vi "TestProgram_SingleStep.vi"() -> ()   [LabVIEW 2011]
uses:
  <instrlib>/Newport ESP301/Newport ESP301.lvlib
panel:
  out "x-y":dbl(graph)
  out "Reduction Ratio":dbl format="%.6g"
  out "Power Status":bool
  out "error out 2":errorcluster
  out "Velocity (units/s)":dbl format="%.4g"
  out "Position (units)":dbl(graph)
  in  "Axis (1)":i32=1
  out "DAC Offset":dbl format="%.6g"
  out "error out":errorcluster
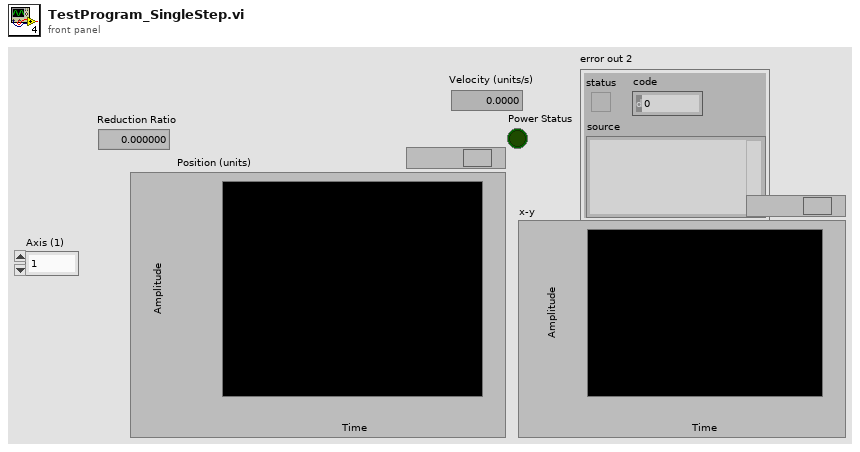
[diagram p1: front panel]
types:
  T1 = enum16{"Trapezoidal Mode", "S-curve Mode", "Jog Mode", "Slave to master's desired position (trajectory)", "Slave to master's actual position (feedback)", "Slave to master's actual velocity for jogging"}
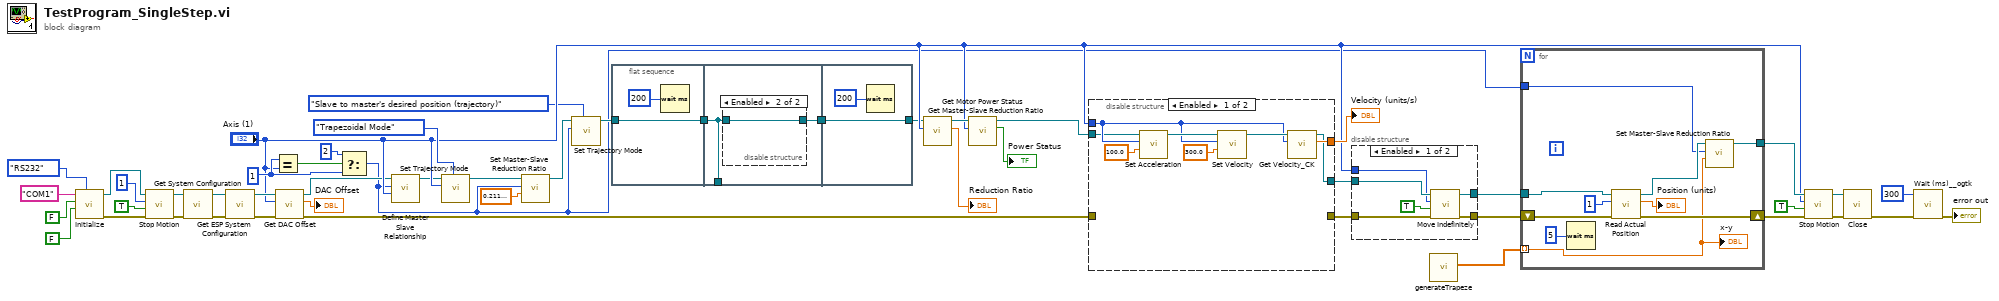
[diagram p0: block diagram]
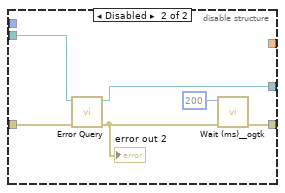
[diagram p2: hidden frame]
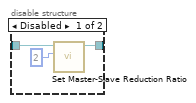
[diagram p3: hidden frame]
diagram:
  w13 = 1 ("x")
  n1 = call <instrlib>:"Initialize.vi"("VISA resource name"="COM1" ("Settings.devport"), "ID Query (True)"=FALSE, "Reset (False)"=FALSE, "Serial Link (RS232)"=enum16{"RS232", "USB"}."RS232") -> ("VISA resource name out"=w45:refnum<visa-resource-name>, "error out"=w43:errorcluster)  [unwired: 5 in]
  n2 = call <instrlib>:"Stop Motion.vi"("error in (no error)"=w43, "Stop all axes (F)"=TRUE, "Axis (1)"=1, "VISA resource name"=w45) -> ("error out"=w41:errorcluster, "VISA resource name out"=w42:refnum<visa-resource-name>)  [unwired: 2 in]
  n3 = call <instrlib>:"Get System Configuration.vi"("error in (no error)"=w41, "VISA resource name"=w42) -> ("error out"=w39:errorcluster, "VISA resource name out"=w40:refnum<visa-resource-name>)  [unwired: 3 in, 1 out]
  n4 = call <instrlib>:"Get ESP System Configuration.vi"("error in (no error)"=w39, "VISA resource name"=w40) -> ("error out"=w36:errorcluster, "VISA resource name out"=w38:refnum<visa-resource-name>)  [unwired: 3 in, 1 out]
  n5 = Equal?(x=w13, y="Axis (1)") -> (x = y?=w15:bool)
  n6 = call <instrlib>:"Get DAC Offset.vi"("error in (no error)"=w36, "Axis (1)"="Axis (1)", "VISA resource name"=w38) -> ("error out"=w24:errorcluster, "DAC Offset"=→"DAC Offset":dbl, "VISA resource name out"=w7:refnum<visa-resource-name>)  [unwired: 2 in]
  n7 = Select(t=2 ("x"), s=w15, f=w13) -> (s? t:f=w2:i32)
  n8 = call <instrlib>:"Define Master Slave Relationship.vi"("Master Axis"="Axis (1)", "Slave Axis"=w2, "VISA resource name"=w7) -> ("VISA resource name out"=w5:refnum<visa-resource-name>)  [unwired: 3 in, 1 out]
  n9 = call <instrlib>:"Set Trajectory Mode.vi"("Trajectory Mode"=T1."Trapezoidal Mode", "Axis (1)"="Axis (1)", "VISA resource name"=w5) -> ("VISA resource name out"=w4:refnum<visa-resource-name>)  [unwired: 4 in, 1 out]
  n10 = call <instrlib>:"Set Master-Slave Reduction Ratio.vi"("Reduction Ratio (0)"=0.21100000000000002, "Axis (1)"=w2, "VISA resource name"=w4) -> ("VISA resource name out"=w3:refnum<visa-resource-name>)  [unwired: 3 in, 1 out]
  n11 = call <instrlib>:"Set Trajectory Mode.vi"("Trajectory Mode"=T1."Slave to master's desired position (trajectory)", "Axis (1)"=w2, "VISA resource name"=w3) -> ("VISA resource name out"=w17:refnum<visa-resource-name>)  [unwired: 4 in, 1 out]
  n12 = flat-sequence {
    tunnel: w17 -> [w52]
    tunnel: [w52] -> w26
    tunnel: [w53] -> _
    tunnel: [w54] -> w27
    tunnel: w26 -> [w53]
    tunnel: [w60] -> w6
    tunnel: w27 -> [w60]
    frame #0 {
      n13 = Wait (ms)(milliseconds to wait=u32 200) -> ()  [unwired: 1 out]
    }
    frame #1 {
      n14 = disable-structure shown="Enabled" {
        disable-tunnel: [w57 w58] -> w54
        disable-tunnel: w53 -> [w55 w58]
        frame Disabled {
          n15 = call <instrlib>:"Set Master-Slave Reduction Ratio.vi"("Axis (1)"=2, "VISA resource name"=w55) -> ("VISA resource name out"=w57:refnum<visa-resource-name>)  [unwired: 4 in, 1 out]
        }
        frame Enabled {
        }
      }
    }
    frame #2 {
      n16 = Wait (ms)(milliseconds to wait=u32 200) -> ()  [unwired: 1 out]
    }
  }
  n17 = call <instrlib>:"Get Master-Slave Reduction Ratio.vi"("Axis (1)"="Axis (1)", "VISA resource name"=w6) -> ("Reduction Ratio"=→"Reduction Ratio":dbl, "VISA resource name out"=w11:refnum<visa-resource-name>)  [unwired: 3 in, 1 out]
  n18 = call <instrlib>:"Get Motor Power Status.vi"("Axis (1)"="Axis (1)", "VISA resource name"=w11) -> ("Power Status"=→"Power Status":bool, "VISA resource name out"=w22:refnum<visa-resource-name>)  [unwired: 3 in, 1 out]
  n19 = disable-structure shown="Enabled" {
    disable-tunnel: [w68 _] -> w35
    disable-tunnel: [w67 w73] -> w34
    disable-tunnel: "Axis (1)" -> [w63 _]
    disable-tunnel: w22 -> [w61 w74]
    disable-tunnel: [_ w70] -> w25
    disable-tunnel: w24 -> [_ w69]
    frame Enabled {
      n20 = call <instrlib>:"Set Acceleration.vi"("Acceleration (0 units/s²)"=100.0, "Axis (1)"=w63, "VISA resource name"=w61) -> ("VISA resource name out"=w64:refnum<visa-resource-name>)  [unwired: 3 in, 1 out]
      n21 = call <instrlib>:"Set Velocity.vi"("Velocity (units/s)"=300.0, "Axis (1)"=w63, "VISA resource name"=w64) -> ("VISA resource name out"=w66:refnum<visa-resource-name>)  [unwired: 3 in, 1 out]
      n22 = call "Get Velocity_CK.vi"("Axis (1)"=w63, "VISA resource name"=w66) -> ("Velocity (units/s)"=w68:dbl, "VISA resource name out"=w67:refnum<visa-resource-name>)  [unwired: 3 in, 1 out]
    }
    frame Disabled {
      n23 = call <instrlib>:"Error Query.vi"("error in (no error)"=w69, "VISA resource name"=w74) -> ("error out"=w72:errorcluster, "VISA resource name out"=w73:refnum<visa-resource-name>)  [unwired: 4 out]
      "error out 2" <- w72
      n24 = call <userlib>:"Wait (ms)__ogtk.vi"("error in (no error)"=w72, "milliseconds to wait"=u32 200) -> ("error out"=w70:errorcluster)  [unwired: 8 in, 1 out]
    }
  }
  "Velocity (units/s)" <- w35
  n25 = disable-structure shown="Enabled" {
    disable-tunnel: w34 -> [w80 w81]
    disable-tunnel: [w78 w81] -> w33
    disable-tunnel: "Axis (1)" -> [w77 _]
    disable-tunnel: w25 -> [w76 _]
    disable-tunnel: [w75 _] -> w23
    frame Enabled {
      n26 = call <instrlib>:"Move Indefinitely.vi"("error in (no error)"=w76, "Move Direction (+)"=TRUE, "Axis (1)"=w77, "VISA resource name"=w80) -> ("error out"=w75:errorcluster, "VISA resource name out"=w78:refnum<visa-resource-name>)  [unwired: 2 in]
    }
    frame Disabled {
    }
  }
  n27 = call "generateTrapeze.vi"() -> ("Ramp Pattern"=w1:dbl[])  [unwired: 11 in]
  n28 = for {
    tunnel: [w84] -> w32
    tunnel: w33 -> [w87]
    shift-right: [w89] -> w30
    shift-left: w23 -> [w88]
    tunnel: w2 -> [w83]
    tunnel: w1 -> [w82] mode=indexing
    n29 = Wait (ms)(milliseconds to wait=u32 5) -> ()  [unwired: 1 out]
    n30 = call <instrlib>:"Read Actual Position.vi"("error in (no error)"=w88, "Axis (1)"=1, "VISA resource name"=w87) -> ("error out"=w89:errorcluster, "Position (units)"=→"Position (units)":dbl, "VISA resource name out"=w85:refnum<visa-resource-name>)  [unwired: 2 in]
    n31 = call <instrlib>:"Set Master-Slave Reduction Ratio.vi"("Reduction Ratio (0)"=w82, "Axis (1)"=w83, "VISA resource name"=w85) -> ("VISA resource name out"=w84:refnum<visa-resource-name>)  [unwired: 3 in, 1 out]
    "x-y" <- w82
  }
  n32 = call <instrlib>:"Stop Motion.vi"("error in (no error)"=w30, "Stop all axes (F)"=TRUE, "Axis (1)"="Axis (1)", "VISA resource name"=w32) -> ("error out"=w28:errorcluster, "VISA resource name out"=w31:refnum<visa-resource-name>)  [unwired: 2 in]
  n33 = call <instrlib>:"Close.vi"("error in (no error)"=w28, "VISA resource name"=w31) -> ("error out"=w20:errorcluster)  [unwired: 9 in]
  n34 = call <userlib>:"Wait (ms)__ogtk.vi"("error in (no error)"=w20, "milliseconds to wait"=u32 300) -> ("error out"=→"error out":errorcluster)  [unwired: 8 in, 1 out]
